vi "ma_SML Averaging (real input, scalar).vi"(3 "reset?":bool, 4 "averaging settings":T1, 5 "x":dbl format="%.2f") -> (0 "data ready?":bool, 1 "averaged sofar":dbl, 2 "y":dbl format="%.2f")   [LabVIEW 2020, in "NI_MAPro.lvlib"]
uses:
  NI_MAPro.lvlib
  ma_sml_Averaging Settings.ctl
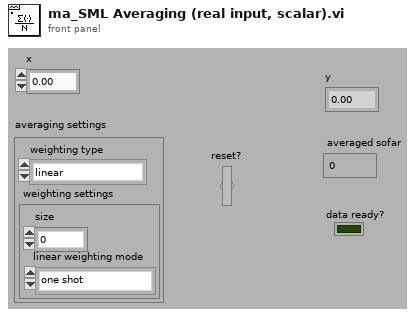
[diagram p1: front panel]
types:
  T1 = typedef "NI_MAPro.lvlib/ma_sml_Averaging Settings.ctl" = cluster{"weighting type":enum16{"linear", "exponential"}, "weighting settings":cluster{"size":dbl, "linear weighting mode":enum16{"one shot", "auto restart one shot", "moving average", "continuous"}}}
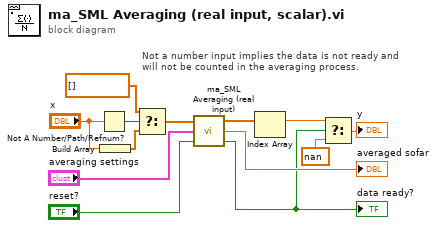
[diagram p0: block diagram]
diagram:
  # "Not a number input implies the data is not ready and \nwill not be counted in the averaging process."
  n1 = Not A Number/Path/Refnum?(number/path/refnum="x") -> (NaN/Path/Refnum?=w13:bool)
  n2 = Build Array("x") -> (w10:dbl[])
  n3 = Select(t=dbl[] [] ("x"), s=w13, f=w10) -> (s? t:f=w12:dbl[])
  n4 = call "ma_SML Averaging (real input).vi"("reset?"="reset?", "averaging settings"="averaging settings", "x"=w12) -> ("data ready?"=w2:bool, "averaged sofar"=→"averaged sofar":dbl, "y"=w6:dbl[])
  "data ready?" <- w2
  n5 = Index Array(array=w6) -> (element=w5:dbl)  [unwired: 1 in]
  n6 = Select(t=w5, s=w2, f=nan) -> (s? t:f=→"y":dbl)
